vi "Changedataconfig.vi"() -> ()   [LabVIEW 2013]
panel:
  in  "OK Button":bool
  out "Input Channel Case":i16
  in  "CH2 Signal Type":bool=TRUE
  in  "CH1 Signal Type":bool=TRUE
  # "Analog"
  # "Counting"
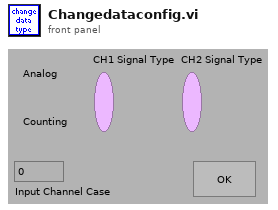
[diagram p1: front panel]
types:
  T1 = cluster{"CH1 AI":tag, "CH1 CI":tag, "CH2 AI":tag, "CH2 CI":tag, "AI X":tag, "AI Y":tag, "AO X-Y":tag, "CH1ST":bool, "CH2ST":bool, "Sigcase":i16, "StageS":i32, "StageL":i32, "data dir":path, "Vp":tag, "Ip":tag, "AO CWlaser":tag, "AO VtoP":tag, "shutter":tag, "488":tag, "532":tag, "640":tag, "LT marker":tag}
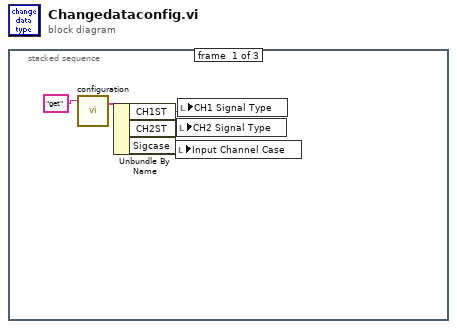
[diagram p0: block diagram]
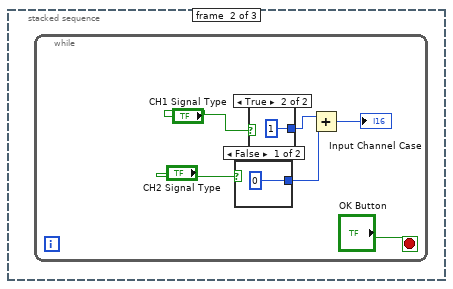
[diagram p2: hidden frame]
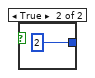
[diagram p3: hidden frame]
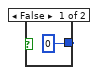
[diagram p4: hidden frame]
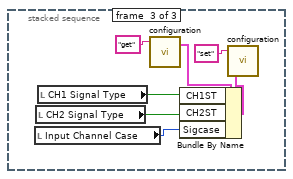
[diagram p5: hidden frame]
diagram:
  n1 = stacked-sequence {
    frame #0 {
      n2 = call "configuration.vi"("command"="get") -> ("config out"=w4:T1)  [unwired: 2 in, 1 out]
      n3 = Unbundle By Name(w4) -> ("CH1ST"=w1:bool, "CH2ST"=w2:bool, "Sigcase"=w3:i16)
      n4 = local write "Input Channel Case"(w3) -> ()
      n5 = local write "CH2 Signal Type"(w2) -> ()
      n6 = local write "CH1 Signal Type"(w1) -> ()
    }
    frame #1 {
      n7 = while {
        stop <- "OK Button" stop-if-true
        n8 = case shown="False" "CH2 Signal Type" {
          tunnel: [i16 0 i16 2] -> w10
          frame False {
          }
          frame True {
          }
        }
        n9 = case shown="True" "CH1 Signal Type" {
          tunnel: [i16 0 i16 1] -> w11
          frame False {
          }
          frame True {
          }
        }
        n10 = Add(x=w11, y=w10) -> (x+y=→"Input Channel Case":i16)
      }
    }
    frame #2 {
      n11 = local read "Input Channel Case"() -> (w16:i16)
      n12 = local read "CH2 Signal Type"() -> (w17:bool)
      n13 = local read "CH1 Signal Type"() -> (w18:bool)
      n14 = call "configuration.vi"("command"="get") -> ("config out"=w20:T1)  [unwired: 2 in, 1 out]
      n15 = Bundle By Name(cluster=w20, "CH1ST"=w18, "CH2ST"=w17, "Sigcase"=w16) -> (w19:T1)
      n16 = call "configuration.vi"("config in"=w19, "command"="set") -> ()  [unwired: 1 in, 2 out]
    }
  }
